vi "NanotecSMCPDDriver.get max velocity.vi"(0 "VISA resource name":refnum<visa-resource-name>, 1 "contollerID":i32=-1, 5 "error in (no error)":errorcluster) -> (14 "VISA resource name out":refnum<visa-resource-name>, 15 "contollerID out":i32=-1, 17 "maxVelocity [Hz]":i32, 19 "error out":errorcluster)   [LabVIEW 2014, in "NanotecSMCPDDriver.lvlib"]
doc: "Gets the maximum velocity (\"stop frequency\") used for the trajectory of a movement."
uses:
  NanotecSMCPDDriver.lvlib
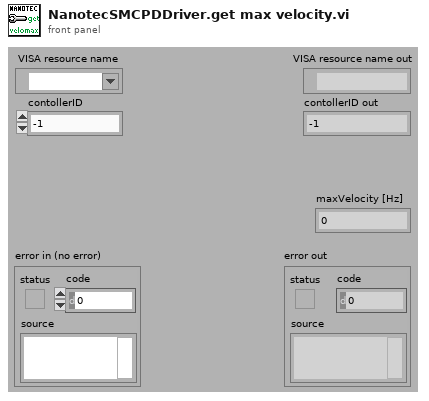
[diagram p1: front panel]
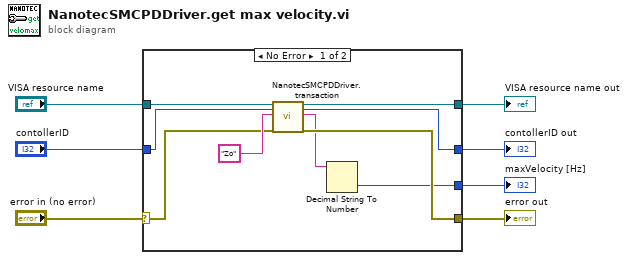
[diagram p0: block diagram]
diagram:
  n1 = case shown="No Error" "error in (no error)" {
    selector: "error in (no error)" -> [w8 w17]
    tunnel: [w15 w19] -> w7
    tunnel: [w14 w17] -> w6
    tunnel: "VISA resource name" -> [w10 w19]
    tunnel: "contollerID" -> [w9 w18]
    tunnel: [w16 w18] -> w3
    tunnel: [w11 _] -> w1
    frame No Error {
      n2 = call "NanotecSMCPDDriver.transaction.vi"("VISAresource"=w10, "contollerID"=w9, "commandString"="Zo", "error in (no error)"=w8) -> ("VISAresource out"=w15:refnum<visa-resource-name>, "contollerID out"=w16:i32, "response"=w12:string, "error out"=w14:errorcluster)  [unwired: 10 in, 2 out]
      n3 = Decimal String To Number(string=w12) -> (number=w11:i32)  [unwired: 2 in, 1 out]
    }
    frame Error {
    }
  }
  "maxVelocity [Hz]" <- w1
  "VISA resource name out" <- w7
  "error out" <- w6
  "contollerID out" <- w3
